vi "Create Framework Configuration.vi"(11 "Plugins":T3(array[cluster])=[{"plugin class"="udp", "channel count per transfer"=100, "transfers per group"=10, "group configs"=[{"direction"=enum."Tx", "timing"={"Decimation"=10, "Offset"=0}}, {"direction"=enum."Rx", "timing"={"Decimation"=10, "Offset"=0}}], "plugin timing"={"Decimation"=10, "Offset"=0}}]) -> (3 "Framework Configuration":T4)   [LabVIEW 2017]
uses:
  DSF.Shared.Refactor.Typedefs.Framework Configuration.Aggregate.ctl
  DSF.Shared.Refactor.Typedefs.Plugin Configuration.Aggregate.ctl
  DSF.Shared.Typedefs.Cycle Timing Factors.ctl
  DSF.Shared.Refactor.Typedefs.Transfer Group Configuration.Aggregate.ctl
  DSF.Shared.Typedefs.Direction.ctl
  DSF.Shared.Refactor.Typedefs.Transfer Configuration.ctl
  DSF.Shared.Typedefs.Byte Order.ctl
  DSF.Shared.Refactor.Typedefs.Channel Array Configuration.ctl
  DSF.Shared.Typedefs.Data Type.ctl
  DSF.Shared.lvlib
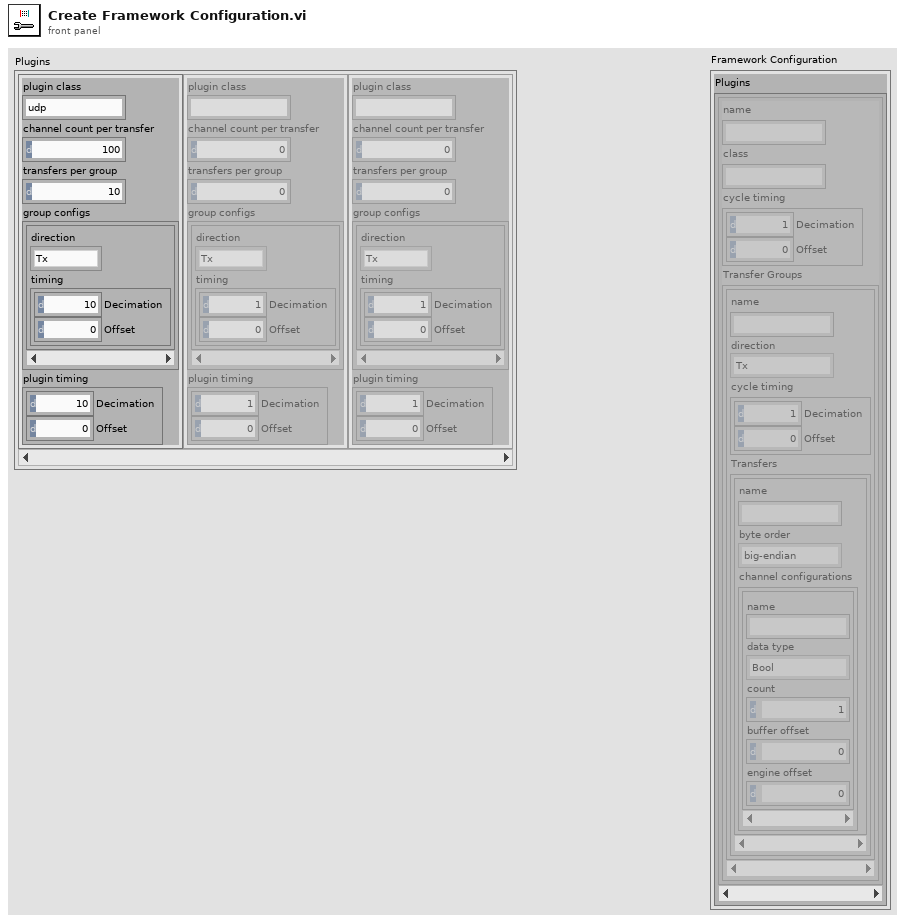
[diagram p1: front panel]
types:
  T1 = typedef "DSF.Shared.lvlib/DSF.Shared.Typedefs.Direction.ctl" = enum8{"Tx", "Rx"}
  T2 = typedef "DSF.Shared.lvlib/DSF.Shared.Typedefs.Cycle Timing Factors.ctl" = cluster{"Decimation":u64, "Offset":u64}
  T3 = cluster{"plugin class":string, "channel count per transfer":i32, "transfers per group":i32, "group configs":cluster{"direction":T1, "timing":T2}[], "plugin timing":T2}[]
  T4 = typedef "DSF.Shared.lvlib/DSF.Shared.Refactor.Typedefs.Framework Configuration.Aggregate.ctl" = cluster{"Plugins":T5[]}
  T5 = typedef "DSF.Shared.lvlib/DSF.Shared.Refactor.Typedefs.Plugin Configuration.Aggregate.ctl" = cluster{"name":string, "class":string, "cycle timing":T2, "Transfer Groups":T6[]}
  T6 = typedef "DSF.Shared.lvlib/DSF.Shared.Refactor.Typedefs.Transfer Group Configuration.Aggregate.ctl" = cluster{"name":string, "direction":T1, "cycle timing":T2, "Transfers":T7[]}
  T7 = typedef "DSF.Shared.lvlib/DSF.Shared.Refactor.Typedefs.Transfer Configuration.ctl" = cluster{"name":string, "byte order":T8, "channel configurations":T9[]}
  T8 = typedef "DSF.Shared.lvlib/DSF.Shared.Typedefs.Byte Order.ctl" = enum8{"big-endian", "little-endian"}
  T9 = typedef "DSF.Shared.lvlib/DSF.Shared.Refactor.Typedefs.Channel Array Configuration.ctl" = cluster{"name":string, "data type":T10, "count":u64, "buffer offset":u64, "engine offset":u64}
  T10 = typedef "DSF.Shared.lvlib/DSF.Shared.Typedefs.Data Type.ctl" = enum8{"Bool", "SGL", "DBL", "I8", "I16", "I32", "I64", "U8", "U16", "U32", "U64"}
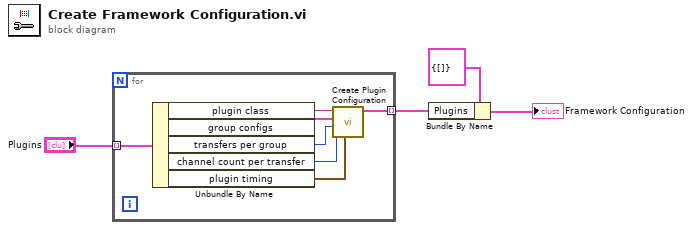
[diagram p0: block diagram]
diagram:
  n1 = for {
    tunnel: [w11] -> w3 mode=indexing
    tunnel: "Plugins" -> [w10] mode=indexing
    n2 = Unbundle By Name(w10) -> ("plugin class"=w9:string, "group configs"=w7:cluster{"direction":T1, "timing":T2}[], "transfers per group"=w6:i32, "channel count per transfer"=w5:i32, "plugin timing"=w8:T2)
    n3 = call "Create Plugin Configuration.vi"("plugin timing"=w8, "channel count per transfer"=w5, "transfers per group"=w6, "group configs"=w7, "plugin class"=w9) -> ("plugin configuration"=w11:T5)  [unwired: 6 in]
  }
  n4 = Bundle By Name(cluster=T4 {"Plugins"=[]} ("Framework Configuration"), "Plugins"=w3) -> (→"Framework Configuration":T4)
